vi "UIRef.vi"(8 "error in":errorcluster, 11 "node in":refnum<class "RunTimeMenuItem.lvclass">) -> (0 "error out":errorcluster, 2 "VI refnum":refnum<vi>, 3 "node out":refnum<class "RunTimeMenuItem.lvclass">)   [LabVIEW 2015, in "RunTimeMenuItem.lvclass"]
doc: "Stores the static reference to the UI of the node."
uses:
  RunTimeMenuItem.lvclass
  RunTimeMenuUI.vi
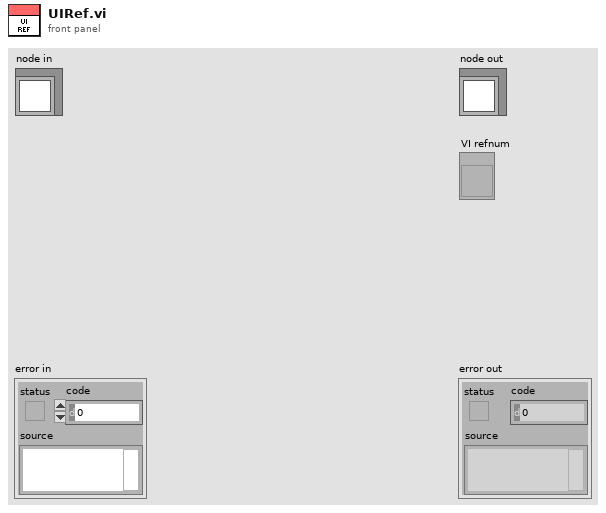
[diagram p1: front panel]
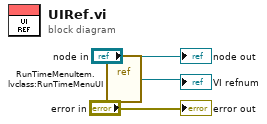
[diagram p0: block diagram]
diagram:
  n1 = vi-ref "RunTimeMenuItem.lvclass:RunTimeMenuUI.vi"() -> (→"VI refnum":refnum<vi>)
  "error out" <- "error in"
  "node out" <- "node in"
